vi "ReadPersistentConfiguration.vi"(8 "ErrorIn":errorcluster, 10 "DataIn":variant, 11 "TemplateGUITAFIn":refnum<class "TemplateGUITAF.lvclass">) -> (0 "ErrorOut":errorcluster, 2 "DataOut":variant, 3 "TemplateGUITAFOut":refnum<class "TemplateGUITAF.lvclass">)   [LabVIEW 2021, in "TemplateGUITAF.lvlib" / "TemplateGUITAF.lvclass"]
uses:
  TemplateGUITAF.lvclass
  TemplateGUITAF.lvclass/TemplateGUITAF.ctl
  C:/Localdata/Projects/TriekselSoft/TriekselsoftApplicationFramework/Source/.Externals/Library_YAF/YAFTAF/YAFTAF.lvclass
  C:/Localdata/Projects/TriekselSoft/TriekselsoftApplicationFramework/Source/.Externals/Library_YAF/YActor/YActor.lvclass
  C:/Localdata/Projects/TriekselSoft/TriekselsoftApplicationFramework/Source/.Externals/Interface_UserInterface_IFrontPanel/IFrontPanel/IFrontPanel.lvclass
  C:/Localdata/Projects/TriekselSoft/TriekselsoftApplicationFramework/Source/IInterface/IInterface.lvclass
  C:/Localdata/Projects/TriekselSoft/TriekselsoftApplicationFramework/Source/.Externals/Interface_Object_ICreateDestroy/ICreateDestroy/ICreateDestroy.lvclass
  C:/Localdata/Projects/TriekselSoft/TriekselsoftApplicationFramework/Source/.Externals/Interface_Object_IPersistentData/IPersistentData/IPersistentData.lvclass
  C:/Localdata/Projects/TriekselSoft/TriekselsoftApplicationFramework/Source/.Externals/Interface_TAF_ITAFObject/ITAFObject/ITAFObject.lvclass
  C:/Localdata/Projects/TriekselSoft/TriekselsoftApplicationFramework/Source/TemplateGUIYAF/TemplateGUITAF/TemplateGUITAF.lvclass
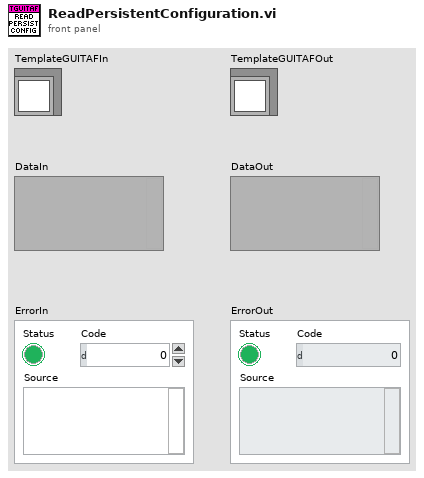
[diagram p1: front panel]
types:
  T1 = cluster{"scaleFactor":dbl, "minNeighbors":i32, "Color":dbl, "Size":cluster{"height":i32, "width":i32}}
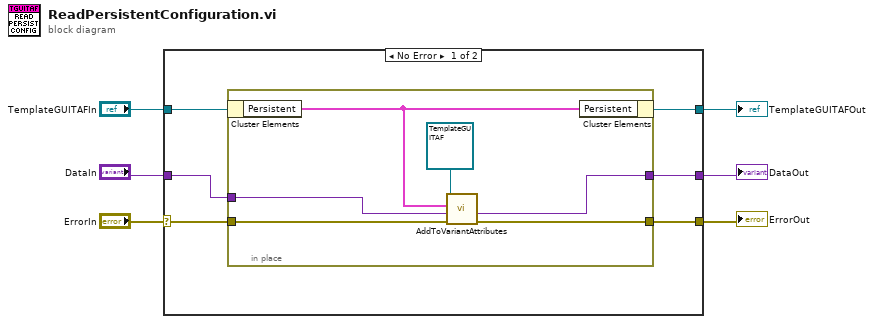
[diagram p0: block diagram]
diagram:
  n1 = case shown="No Error" "ErrorIn" {
    selector: "ErrorIn" -> [w12 w21]
    tunnel: [w11 w21] -> w5
    tunnel: [w7 w20] -> w3
    tunnel: "TemplateGUITAFIn" -> [w10 w20]
    tunnel: "DataIn" -> [w9 w19]
    tunnel: [w8 w19] -> w1
    frame No Error {
      n2 = in-place {
        in-place-border: [w17] -> w11
        in-place-border: w9 -> [w16]
        in-place-border: [w15] -> w8
        in-place-border: w12 -> [w18]
        n3 = in-place-cluster #1(w10) -> ("Persistent"=w13:T1)
        n4 = call "AddToVariantAttributes.vi"("ErrorIn"=w18, "DataInIn"=w16, "PersistentData"=w13, "Object"=refnum<class "TemplateGUITAF.lvclass"> refnum ("ApplicationGUI2")) -> ("ErrorOut"=w17:errorcluster, "DataInOut"=w15:variant)  [unwired: 6 in]
        n5 = in-place-cluster #1("Persistent"=w13) -> (w7:refnum<class "TemplateGUITAF.lvclass">)
      }
    }
    frame Error {
    }
  }
  "ErrorOut" <- w5
  "TemplateGUITAFOut" <- w3
  "DataOut" <- w1
